vi "Pop up.vi"() -> (0 "Continue":bool)   [LabVIEW 2018]
panel:
  in  "Abort":bool
  in  "Continue":bool
  # "WARNING: Are you measuring this tube again?"
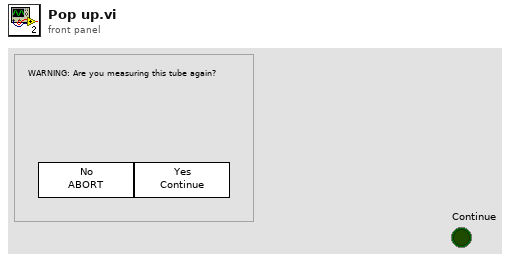
[diagram p1: front panel]
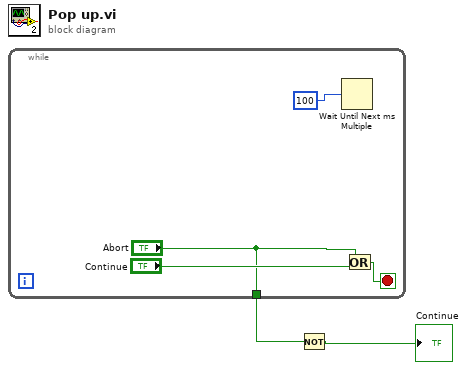
[diagram p0: block diagram]
diagram:
  n1 = while {
    tunnel: ["Abort"] -> w1
    stop <- w6 stop-if-true
    n2 = Wait Until Next ms Multiple(millisecond multiple=u32 100 ("milliseconds to wait")) -> ()  [unwired: 1 out]
    n3 = Or(x="Abort", y="Continue") -> (x .or. y?=w6:bool)
  }
  n4 = Not(x=w1) -> (.not. x?=→"Continue":bool)
